vi "获取标签所有属性.vi"(8 "error in (no error)":errorcluster caption="错误输入（无错误）", 11 "XML Node String In":string caption="XML节点字符串输入") -> (0 "error out":errorcluster, 3 "xml attribute out":string[][](array[string]) caption="xml节点属性", 5 "node name":string caption="节点名称")   [LabVIEW 2017]
panel:
  # "查找元素VI获取的元素名"
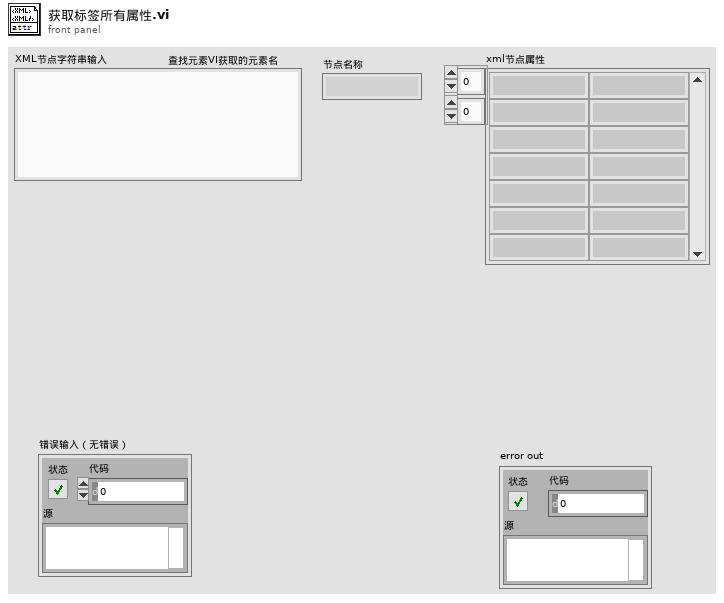
[diagram p1: front panel]
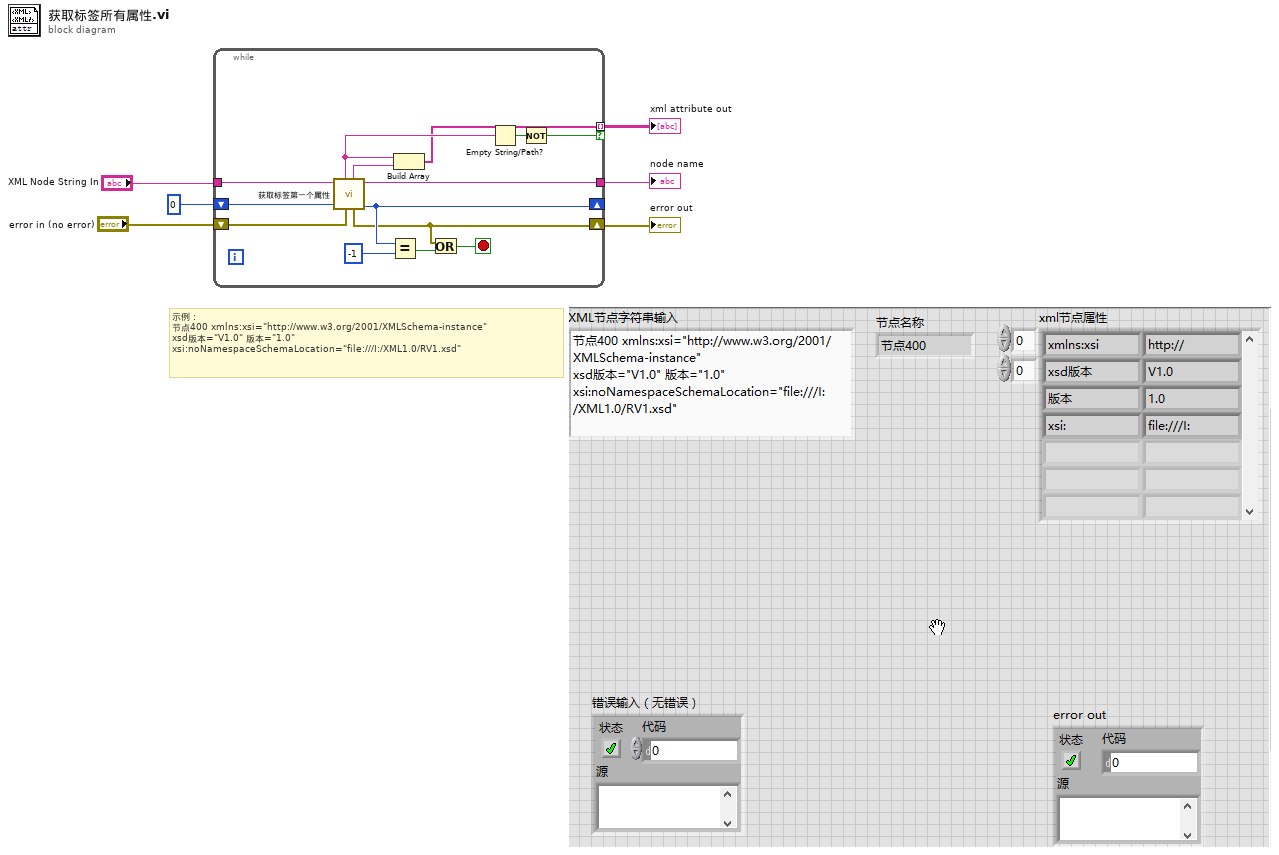
[diagram p0: block diagram]
diagram:
  # "示例：\n节点400 xmlns:xsi=\"http://www.w3.org/2001/XMLSchema-instance\" \nxsd版本=\"V1.0\" 版本=\"1.0\" \nxsi:noNamespaceSchemaLocation=\"file:///I:/XML1.0/RV1.xsd\""
  n1 = while {
    shift-right: [w17] -> _
    shift-left: 0 ("offset past match") -> [w19]
    tunnel: "XML Node String In" -> [w18]
    shift-right: [w13] -> w4
    shift-left: "error in (no error)" -> [w16]
    tunnel: [w10] -> w2 mode=indexing if=w9
    tunnel: [w7] -> w1
    stop <- w14 stop-if-true
    n2 = call "获取标签第一个属性.vi"("error in (no error)"=w16, "offset (0)"=w19, "XML String In"=w18) -> ("offset past match"=w17:i32, "node name"=w7:string, "error out"=w13:errorcluster, "attribute value"=w20:string, "attribute name"=w11:string)  [unwired: 2 in, 2 out]
    n3 = Equal?(x=w17, y=-1) -> (x = y?=w15:bool)
    n4 = Build Array(w11, w20) -> (w10:string[])
    n5 = Or(x=w13, y=w15) -> (x .or. y?=w14:bool)
    n6 = Empty String/Path?(string/path=w11) -> (empty?=w8:bool)
    n7 = Not(x=w8) -> (.not. x?=w9:bool)
  }
  "xml attribute out" <- w2
  "error out" <- w4
  "node name" <- w1
